vi "Raft_wars_Ver3.vi"() -> ()   [LabVIEW 2026]
panel:
  out "x .and. y?":bool
  out "x .or. y?":bool
  out "Numeric 2":i32
  out "Numeric":i32
  out "X-Coordinate":i32
  out "Y-Coordinate":i32
  out "Array":dbl[][](array[numeric])
  in  "Player Ship Inputs":T1(array[cluster]) {"Y-Coordinate" min=0 max=7; "X-Coordinate" min=0 max=7}
  in  "Emergency Stop":bool
  out "Game Status":string
  out "Ships Placed":dbl
  out "Losses":dbl
  out "Computer Hits":dbl
  out "Wins":dbl
  out "Player Hits":dbl
  in  "Attack":bool
  in  "Play Again":bool
  in  "Place Ship":bool
  in  "Attack Y":dbl
  in  "Attack X":dbl
  in  "Ship Y":i32
  in  "Ship X":i32
  out "Computer  Board":u32[][][][][][][][](array[colorbox])
  out "Player Board":u32[][][][][][][][](array[colorbox])
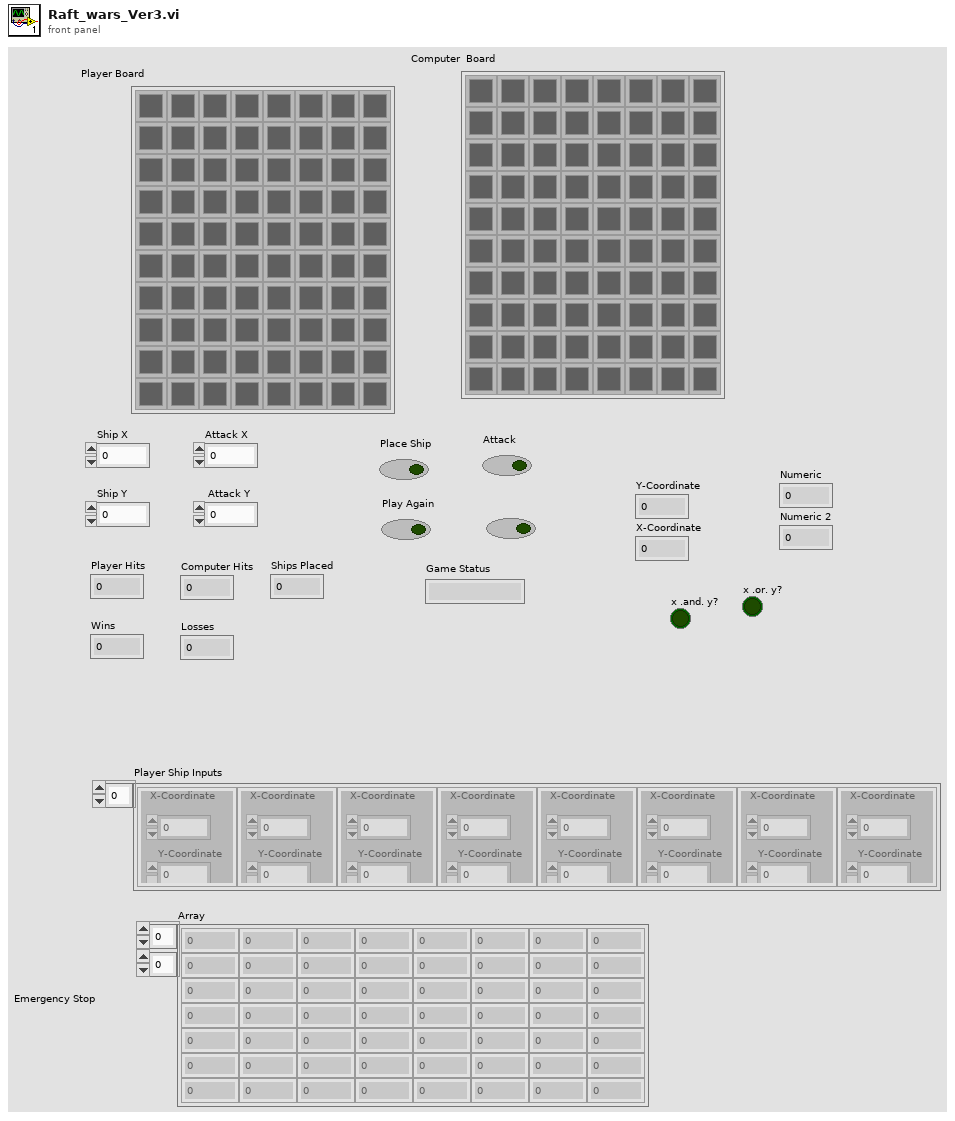
[diagram p1: front panel]
types:
  T1 = cluster{"X-Coordinate":i32, "Y-Coordinate":i32}[]
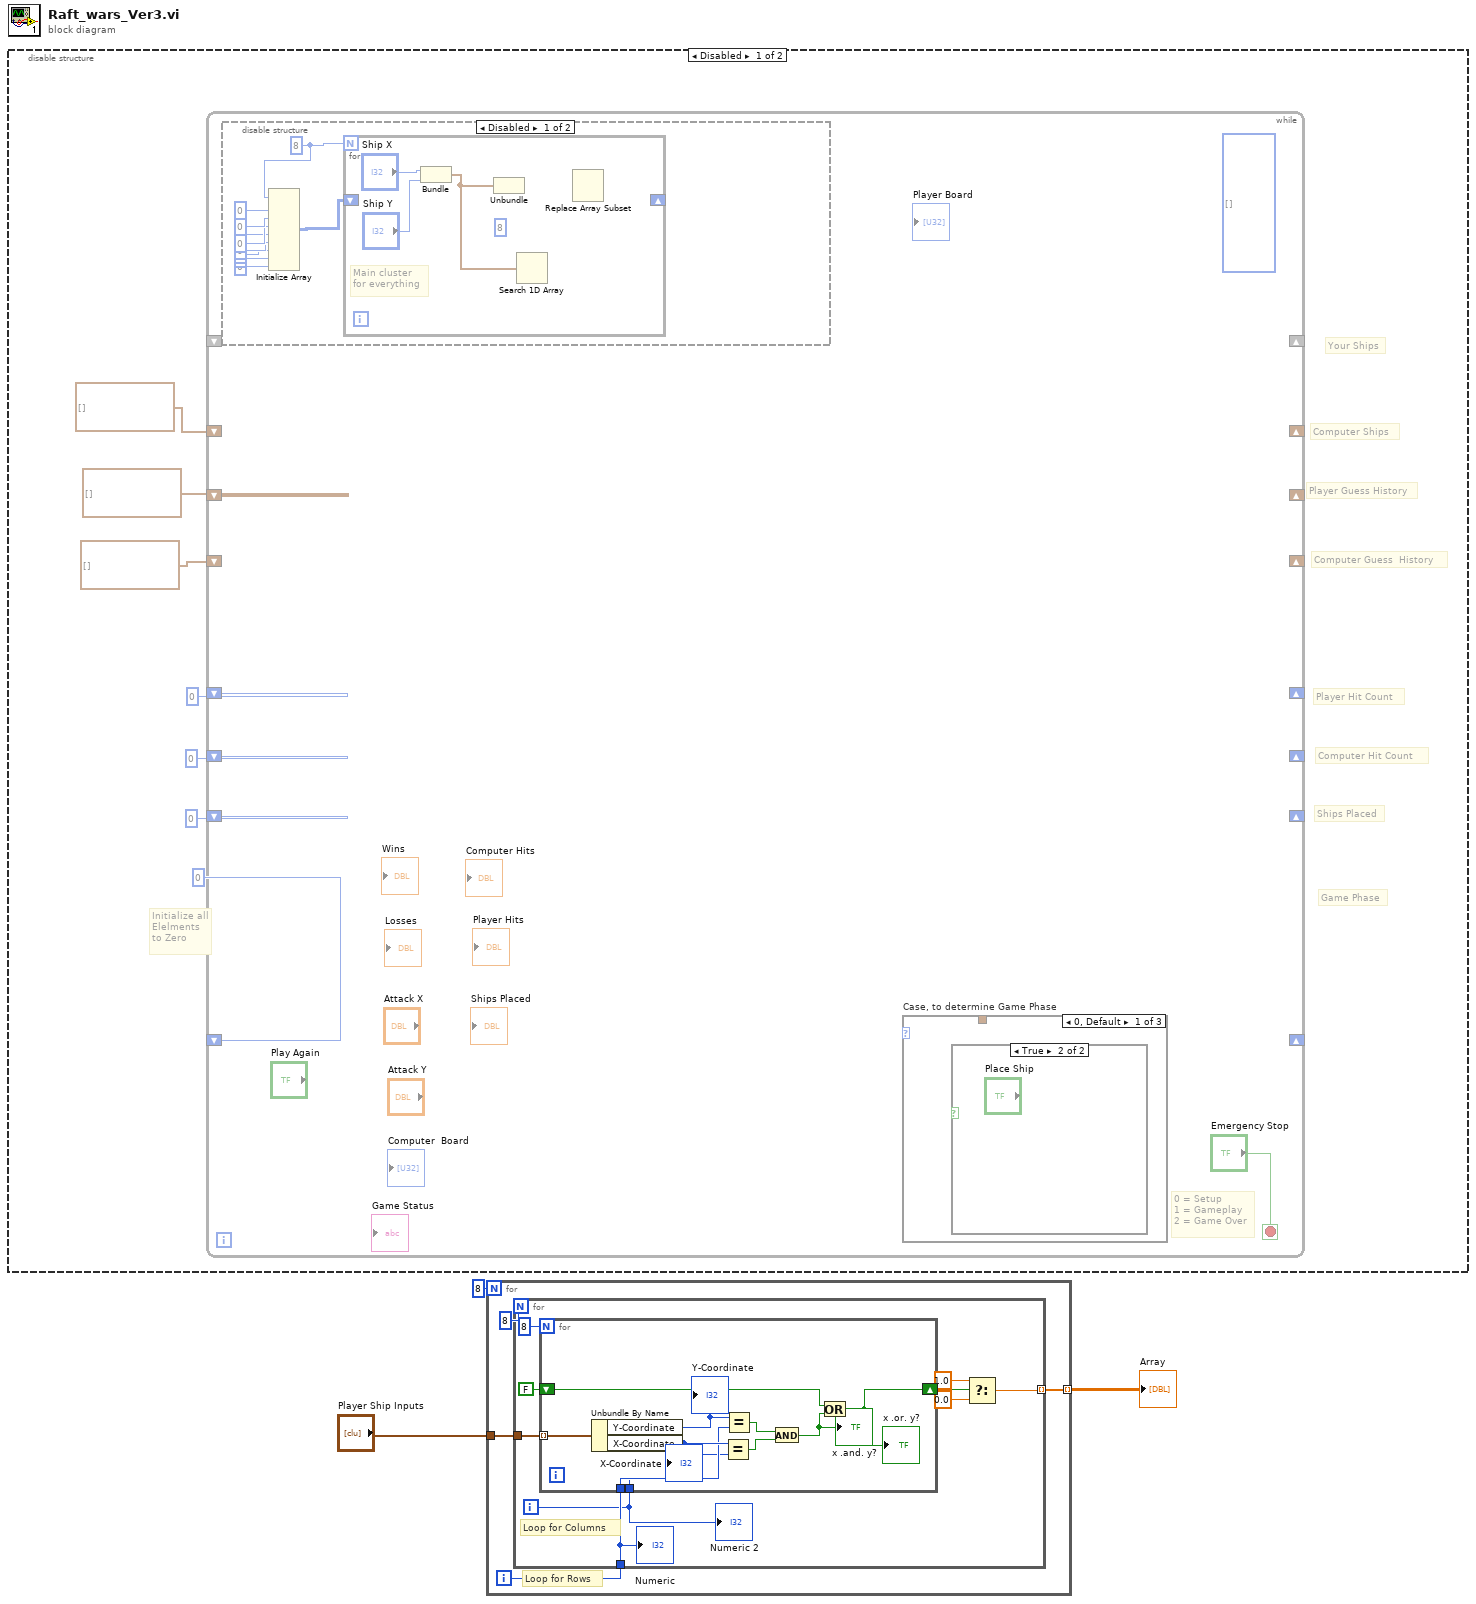
[diagram p0: block diagram]
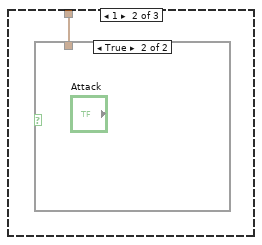
[diagram p4: hidden frame]
diagram:
  n1 = disable-structure shown="Disabled" {
    frame Disabled {
      # "Initialize all\nElelments\nto Zero"
      # "Ships Placed"
      # "Your Ships"
      # "Computer Ships"
      # "Player Guess History"
      # "Computer Guess  History"
      # "Player Hit Count"
      # "Computer Hit Count"
      # "Game Phase"
      n2 = while {
        shift-right: _ -> [_]
        shift-left: _ -> [_]
        shift-right: _ -> [_]
        shift-left: cluster{dbl, dbl}[] [] -> [_]
        shift-right: _ -> [_]
        shift-left: cluster{dbl, dbl}[] [] -> [_]
        shift-right: _ -> [_]
        shift-left: cluster{dbl, dbl}[] [] -> [_]
        shift-right: _ -> [_]
        shift-left: 0 -> [_]
        shift-right: _ -> [_]
        shift-left: 0 -> [_]
        shift-right: _ -> [_]
        shift-left: 0 -> [_]
        shift-right: _ -> [_]
        shift-left: 0 -> [_]
        stop <- "Emergency Stop" stop-if-true
        (unwired) u32[][][][][][][][] [] ("PLayer 1 Board 2")
        # "0 = Setup\n1 = Gameplay\n2 = Game Over"
        n3 = disable-structure shown="Disabled" {
          frame Disabled {
            w20 = 8
            n4 = Initialize Array(w20, 0 ("dimension size"), 0 ("dimension size"), 0 ("dimension size"), 0 ("dimension size"), 0 ("dimension size"), 0 ("dimension size"), 0 ("dimension size"), 0 ("dimension size")) -> (w21:i32[][][][][][][][])
            n5 = for {
              N: w20 -> [_]
              shift-right: _ -> [w22]
              shift-left: w21 -> [_]
              (unwired) 8
              # "Main cluster\nfor everything"
              n6 = Bundle("Ship X"="Ship X", "Ship Y"="Ship Y") -> (w23:cluster{"Ship X":i32, "Ship Y":i32})  [unwired: 1 in]
              n7 = Unbundle(w23) -> ()  [unwired: 2 out]
              n8 = Search 1D Array(element=w23) -> ()  [unwired: 2 in, 1 out]
              n9 = Replace Array Subset() -> ()  [unwired: 3 in, 1 out]
            }
          }
          frame Enabled {
          }
        }
        n10 = case "Case, to determine Game Phase" shown="0, Default" {
          selector: _ -> [_ _ _]
          tunnel: _ -> [_ w26 _]
          frame 0, Default {
            n11 = case shown="True" {
              selector: _ -> [_ _]
              frame False {
              }
              frame True {
              }
            }
          }
          frame 1 {
            n12 = case shown="True" {
              selector: _ -> [_ _]
              tunnel: w26 -> [_ _]
              frame False {
              }
              frame True {
              }
            }
          }
          frame 2 {
          }
        }
      }
    }
    frame Enabled {
    }
  }
  n13 = for {
    N: 8 -> [_]
    tunnel: "Player Ship Inputs" -> [w27]
    tunnel: [w28] -> w3 mode=indexing
    i -> [w29]
    # "Loop for Rows"
    n14 = for {
      N: 8 -> [_]
      tunnel: w29 -> [w39]
      tunnel: [w34] -> w28 mode=indexing
      tunnel: w27 -> [w31]
      i -> [w38]
      # "Loop for Columns"
      n15 = for {
        N: 8 -> [_]
        tunnel: w39 -> [w42]
        tunnel: w38 -> [w41]
        shift-right: [w43] -> w37
        shift-left: FALSE -> [w44]
        tunnel: w31 -> [w40] mode=indexing
        n16 = Unbundle By Name(w40) -> ("Y-Coordinate"=w48:i32, "X-Coordinate"=w49:i32)
        "Y-Coordinate" <- w48
        "X-Coordinate" <- w49
        n17 = Equal?(x=w49, y=w41) -> (x = y?=w46:bool)
        n18 = Equal?(x=w48, y=w42) -> (x = y?=w47:bool)
        n19 = And(x=w47, y=w46) -> (x .and. y?=w45:bool)
        "x .and. y?" <- w45
        n20 = Or(x=w44, y=w45) -> (x .or. y?=w43:bool)
        "x .or. y?" <- w43
      }
      n21 = Select(t=1.0, s=w37, f=0.0) -> (s? t:f=w34:dbl)
      "Numeric" <- w39
      "Numeric 2" <- w38
    }
  }
  "Array" <- w3
